vi "Self test.vi"(8 "error in (no error)":errorcluster, 11 "Accelerometer":T1) -> (0 "error out":errorcluster, 1 "accel self test":dbl[](array[numeric]), 2 "gyro self test":dbl[](array[numeric]), 3 "Accelerometer out":T1, 4 "good":bool)   [LabVIEW 2013]
doc: "Use this template to build a VI to use as a subVI."
uses:
  AccelerometerSPI.ctl
  <vilib>/ni845x/ni845x.llb/ni845xControl.ctl
  <vilib>/ni845x/ni845x.llb/ni845xSpiConfiguration.ctl
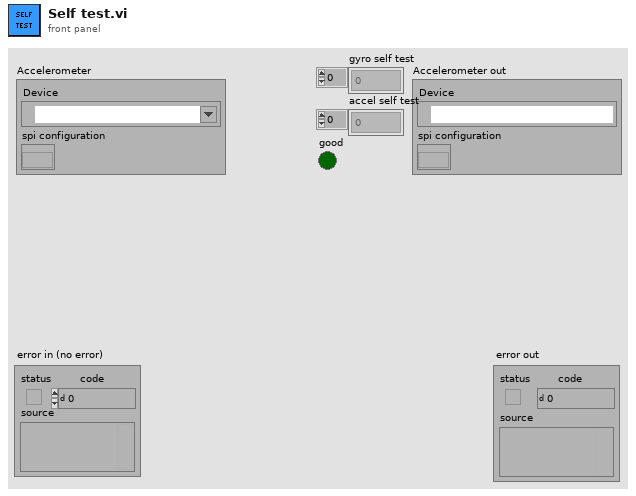
[diagram p1: front panel]
types:
  T1 = typedef "AccelerometerSPI.ctl" = cluster{"Device":T2, "spi configuration":T3}
  T2 = typedef "ni845xControl.ctl" = refnum<k21>
  T3 = typedef "ni845xSpiConfiguration.ctl" = refnum<k20>
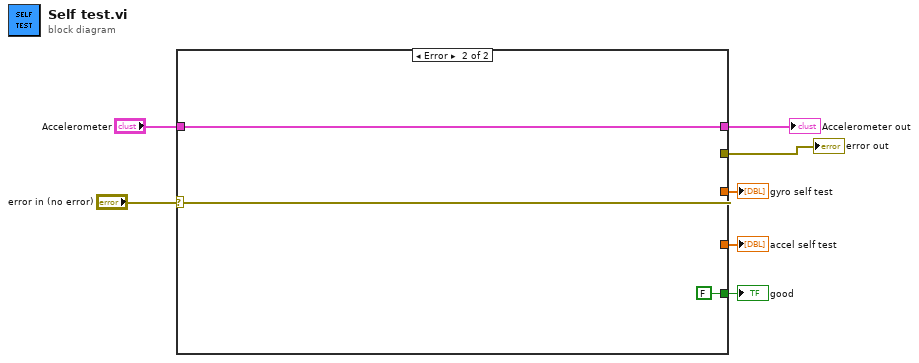
[diagram p0: block diagram]
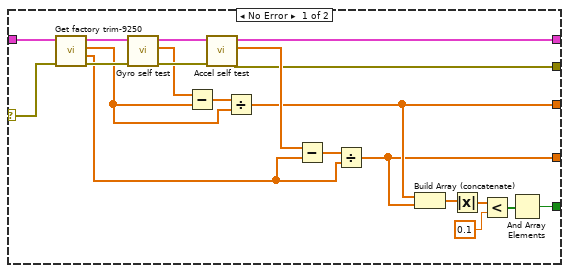
[diagram p2: hidden frame]
diagram:
  n1 = case shown="Error" "error in (no error)" {
    selector: "error in (no error)" -> [w15 w31]
    tunnel: [w16 w31] -> w6
    tunnel: "Accelerometer" -> [w28 w30]
    tunnel: [w17 w30] -> w4
    tunnel: [w11 _] -> w3
    tunnel: [w10 _] -> w2
    tunnel: [w8 FALSE] -> w1
    frame No Error {
      n2 = call "Get factory trim-9250.vi"("error in (no error)"=w15, "Accelerometer"=w28) -> ("error out"=w26:errorcluster, "Accel trim"=w18:dbl[], "Gyro trim"=w21:dbl[], "Accelerometer out"=w27:T1)  [unwired: 6 in]
      n3 = call "Gyro self test.vi"("error in (no error)"=w26, "Accelerometer"=w27) -> ("error out"=w24:errorcluster, "gyro self test"=w23:dbl[], "Accelerometer out"=w25:T1)  [unwired: 7 in]
      n4 = Subtract(x=w23, y=w21) -> (x-y=w22:dbl[])
      n5 = call "Accel self test.vi"("error in (no error)"=w24, "Accelerometer"=w25) -> ("error out"=w16:errorcluster, "accel self test"=w19:dbl[], "Accelerometer out"=w17:T1)  [unwired: 7 in]
      n6 = Divide(x=w22, y=w21) -> (x/y=w11:dbl[])
      n7 = Subtract(x=w19, y=w18) -> (x-y=w20:dbl[])
      n8 = Divide(x=w20, y=w18) -> (x/y=w10:dbl[])
      n9 = Build Array (concatenate)(w11, w10) -> (w12:dbl[])
      n10 = Absolute Value(x=w12) -> (abs(x)=w13:dbl[])
      n11 = Less?(x=w13, y=0.1) -> (x < y?=w9:bool[])
      n12 = And Array Elements(Boolean array=w9) -> (logical AND=w8:bool)
    }
    frame Error {
    }
  }
  "error out" <- w6
  "Accelerometer out" <- w4
  "gyro self test" <- w3
  "accel self test" <- w2
  "good" <- w1
